vi "Brent with Derivatives Prep.vi"(0 "result":dbl[](array[numeric]) format="%.2f", 4 "values":T1 {"c (start)" format="%.2f"; "b (start)" format="%.2f"; "a (start)" format="%.2f"}, 5 "accuracy":dbl format="%.2f", 6 "table":i32[][](array[numeric]), 7 "inner case":bool, 8 "list of variables":i32[](array[numeric]), 9 "outer case":bool) -> (1 "error":i32, 2 "f(minimum)":dbl format="%.2f", 3 "minimum":dbl format="%.2f")   [LabVIEW 2020, in "NI_Gmath.lvlib"]
uses:
  <vilib>/gmath/NI_Gmath.lvlib
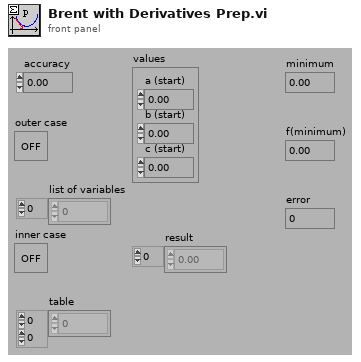
[diagram p1: front panel]
types:
  T1 = cluster{"a (start)":dbl, "b (start) ":dbl, "c (start)":dbl}
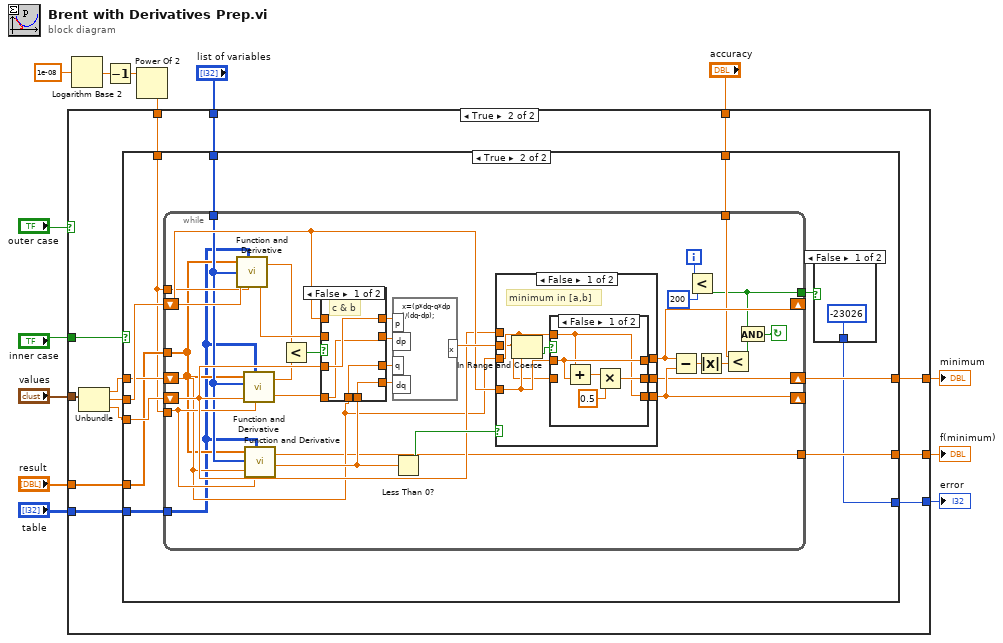
[diagram p0: block diagram]
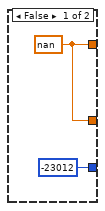
[diagram p2: hidden frame]
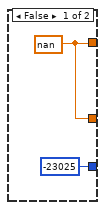
[diagram p3: hidden frame]
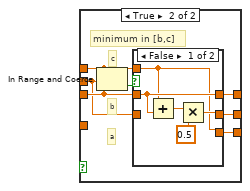
[diagram p6: hidden frame]
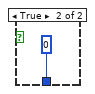
[diagram p8: hidden frame]
diagram:
  n1 = Logarithm Base 2(1:1e-08) -> (0:w3:dbl)
  n2 = Decrement(x=w3) -> (x-1=w2:dbl)
  n3 = Power Of 2(x=w2) -> (2^x=w1:dbl)
  n4 = case shown="True" "outer case" {
    tunnel: [w16 w29] -> w7
    tunnel: [w16 w28] -> w6
    tunnel: "inner case" -> [_ w27]
    tunnel: "accuracy" -> [_ w26]
    tunnel: [-23012 w25] -> w10
    tunnel: "list of variables" -> [_ w24]
    tunnel: "table" -> [_ w23]
    tunnel: "result" -> [_ w22]
    tunnel: "values" -> [_ w21]
    tunnel: w1 -> [_ w17]
    frame False {
      w16 = nan
    }
    frame True {
      n5 = Unbundle(w21) -> ("a (start)"=w20:dbl, "b (start)"=w19:dbl, "c (start)"=w18:dbl)
      n6 = case shown="True" w27 {
        tunnel: w19 -> [_ w43]
        tunnel: w20 -> [_ w42]
        tunnel: w18 -> [_ w41]
        tunnel: [w31 w40] -> w28
        tunnel: [w31 w39] -> w29
        tunnel: w26 -> [_ w38]
        tunnel: [-23025 w36] -> w25
        tunnel: w24 -> [_ w35]
        tunnel: w23 -> [_ w34]
        tunnel: w22 -> [_ w33]
        tunnel: w17 -> [_ w32]
        frame False {
          w31 = nan
        }
        frame True {
          n7 = while {
            tunnel: w33 -> [w45]
            tunnel: w34 -> [w44]
            tunnel: w35 -> [w46]
            tunnel: [w49] -> w37
            tunnel: w38 -> [w52]
            tunnel: [w53] -> w39
            tunnel: w32 -> [w58]
            tunnel: w32 -> [w62]
            shift-left: w41 -> [w60]
            shift-right: [w68] -> _
            shift-left: w42 -> [w57]
            shift-right: [w54] -> w40
            shift-left: w43 -> [w64]
            shift-right: [w69] -> _
            i -> [w51]
            stop <- w47 continue-if-true
            n8 = call <vilib>:"Function and Derivative.vi"("result"=w45, "table"=w44, "list of variables"=w46, "x"=w64, "(x+h)-x"=w62) -> ("f(x)"=w56:dbl, "df(x)/dx"=w63:dbl)
            n9 = call <vilib>:"Function and Derivative.vi"("result"=w45, "table"=w44, "list of variables"=w46, "x"=w60, "(x+h)-x"=w58) -> ("f(x)"=w55:dbl, "df(x)/dx"=w61:dbl)
            n10 = call <vilib>:"Function and Derivative.vi"("result"=w45, "table"=w44, "list of variables"=w46, "x"=w57, "(x+h)-x"=w58) -> ("f(x)"=w53:dbl, "df(x)/dx"=w59:dbl)
            n11 = Less?(x=w56, y=w55) -> (x < y?=w75:bool)
            n12 = case shown="False" w75 {
              tunnel: w60 -> [w77 _]
              tunnel: w59 -> [w78 w80]
              tunnel: w61 -> [w76 _]
              tunnel: w63 -> [_ w82]
              tunnel: w64 -> [_ w83]
              tunnel: [w77 w83] -> w74
              tunnel: [w76 w82] -> w73
              tunnel: w57 -> [w79 w81]
              tunnel: [w79 w81] -> w72
              tunnel: [w78 w80] -> w71
              frame False {
                # "c & b"
              }
              frame True {
                # "a & b"
              }
            }
            n13 = formula code="x=(p*dq-q*dp)/(dq-dp);"("p"=w74, "q"=w72, "dp"=w73, "dq"=w71) -> ("x"=w66:dbl)
            n14 = Less Than 0?(x=w59) -> (x < 0?=w70:bool)
            n15 = case shown="False" w70 {
              tunnel: w66 -> [w86 w102]
              tunnel: w57 -> [w89 w104]
              tunnel: w60 -> [_ w100]
              tunnel: w64 -> [w87 _]
              tunnel: [w88 w103] -> w69
              tunnel: [w85 w101] -> w54
              tunnel: [w84 w99] -> w68
              frame False {
                # "minimum in [a,b]"
                n16 = In Range and Coerce(upper limit=w89, x=w86, lower limit=w87) -> (In Range?=w90:bool)  [unwired: 1 out]
                n17 = case shown="False" w90 {
                  tunnel: w87 -> [w93 w98]
                  tunnel: [w93 w98] -> w88
                  tunnel: w86 -> [_ w97]
                  tunnel: [w92 w97] -> w85
                  tunnel: w89 -> [w91 w96]
                  tunnel: [w91 w96] -> w84
                  frame False {
                    n18 = Add(x=w91, y=w93) -> (x+y=w95:dbl)
                    n19 = Multiply(x=w95, y=0.5) -> (x*y=w92:dbl)
                  }
                  frame True {
                  }
                }
              }
              frame True {
                # "b"
                # "c"
                # "a"
                # "minimum in [b,c]"
                n20 = In Range and Coerce(upper limit=w100, x=w102, lower limit=w104) -> (In Range?=w105:bool)  [unwired: 1 out]
                n21 = case shown="False" w105 {
                  tunnel: w104 -> [w108 w113]
                  tunnel: [w108 w113] -> w103
                  tunnel: w102 -> [_ w112]
                  tunnel: [w107 w112] -> w101
                  tunnel: w100 -> [w106 w111]
                  tunnel: [w106 w111] -> w99
                  frame False {
                    n22 = Add(x=w106, y=w108) -> (x+y=w110:dbl)
                    n23 = Multiply(x=w110, y=0.5) -> (x*y=w107:dbl)
                  }
                  frame True {
                  }
                }
              }
            }
            n24 = Subtract(x=w69, y=w68) -> (x-y=w67:dbl)
            n25 = Less?(x=w51, y=200) -> (x < y?=w49:bool)
            n26 = Absolute Value(x=w67) -> (abs(x)=w65:dbl)
            n27 = Less?(x=w52, y=w65) -> (x < y?=w48:bool)
            n28 = And(x=w49, y=w48) -> (x .and. y?=w47:bool)
          }
          n29 = case shown="False" w37 {
            tunnel: [-23026 0] -> w36
            frame False {
            }
            frame True {
            }
          }
        }
      }
    }
  }
  "error" <- w10
  "f(minimum)" <- w7
  "minimum" <- w6
